vi "Create Mode.vi"   [LabVIEW 2017, in "Scan Engine Scripting.lvlib"]
uses:
  Scan Engine Scripting.lvlib
  Digital Output Mode/Digital Output Mode.lvclass
  Digital Input Mode/Digital Input Mode.lvclass
  PWM Mode/PWM Mode.lvclass
  Analog Input Mode/Analog Input Vrms Mode/Analog Input Mode.lvclass
  Analog Input Vrms Mode/Analog Input Vrms Mode.lvclass
  Mode/Mode.lvclass
  Counter Driven Output Mode/Counter Driven Output Mode.lvclass
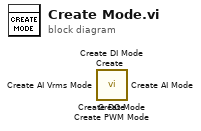
[diagram p0: block diagram]
diagram:
  n1 = call-dynamic "Create.vi"() -> ()  [unwired: 9 in, 3 out]
  n2 = call-dynamic "Create.vi"() -> ()  [unwired: 9 in, 3 out]
  n3 = call "Create AI Vrms Mode.vi"() -> ()  [unwired: 9 in, 3 out]
  n4 = call "Create AI Mode.vi"() -> ()  [unwired: 9 in, 3 out]
  n5 = call "Create PWM Mode.vi"() -> ()  [unwired: 9 in, 3 out]
  n6 = call "Create DI Mode.vi"() -> ()  [unwired: 9 in, 3 out]
  n7 = call "Create DO Mode.vi"() -> ()  [unwired: 9 in, 3 out]
